vi "SemiProbe.vi"() -> ()   [LabVIEW 2019, in "SemiProbe.lvclass"]
uses:
  SemiProbe.lvclass
panel:
  in  "SemiProbe Probestation configuration":T1={"SP Local"=FALSE, "SP Min Usable Z"=0.0, "SP REMOTE Comm Parameters"={"SemiProbe VISA"="", "write delay(ms)"=500, "buffer is full loop multiplicity"=10, "read threshold check rate (ms)"=50}, "SP Comm Params"={"LF as Return EOL"=TRUE, "SP Error Debug"=FALSE}, "SP LOCAL Comm Parameters"={"address"="localhost", "port"=5050, "SP TCP Cnx ID"=refnum, "mode (standard)"=enum."Immediate", "bytes to read"=300, "timeout (ms)"=1000000}, "SP Operation Parameters"={"SP Load Less Than Thr?"=TRUE, "SP Load Threshold (um)"=4800.0, "SP Current Location"={"X (um)"=20.0, "Y (um)"=20.0, "Z (um)"=20.0, "T (degree)"=20.0}, "SP Chuck Speeds"={"XY Speed (10-100%)"=10.0, "Z Speed (10-100%)"=10.0, "T Speed (10-100%)"=10.0}, "Manual Step Parameters"={"Step in X"=FALSE, "X S-Speed [µm/step]"=5.0, "Step in Y"=FALSE, "Y S-Speed [µm/step]"=5.0, "Step in Z"=FALSE, "Z S-Speed [µm/step]"=5.0, "Step in T"=FALSE, "T S-Speed [mdegree/step]"=5.0, "X Increase"=TRUE, "Y Increase?"=TRUE, "Z Increase?"=TRUE, "T Increase?"=TRUE}, "Z Stepper"={"UP/DOWN"=FALSE, "UP/DOWN Speed [µm/step]"=20, "SP Z Step"=FALSE}, "Z Heights Set"=FALSE, "SP Contact Search"={"Contact Circuit"=enum."1", "Speed [1000-10000]"=1000.0, "Start Height [µm]"=0.0, "Search Band [µm]"=100.0, "Overdrive [µm]"=30.0}, "Separation Distance [µm]"=0, "Contact Height [µm]"=0, "Use Overdrive?"=FALSE, "Touchdown method"=enum."no feedback", "Arduino Edgesense params"={"touchdown height [µm]"=0, "search band [µm]"=100, "speed [µm/step]"=10, "overdrive [µm]"=30}}} {"SP Operation Parameters"."SP Contact Search"."Speed [1000-10000]" min=1000 max=10000; "SP Operation Parameters"."SP Load Threshold (um)" format="%#_6f"}
  # "Of value set in the SP Navigation panel."
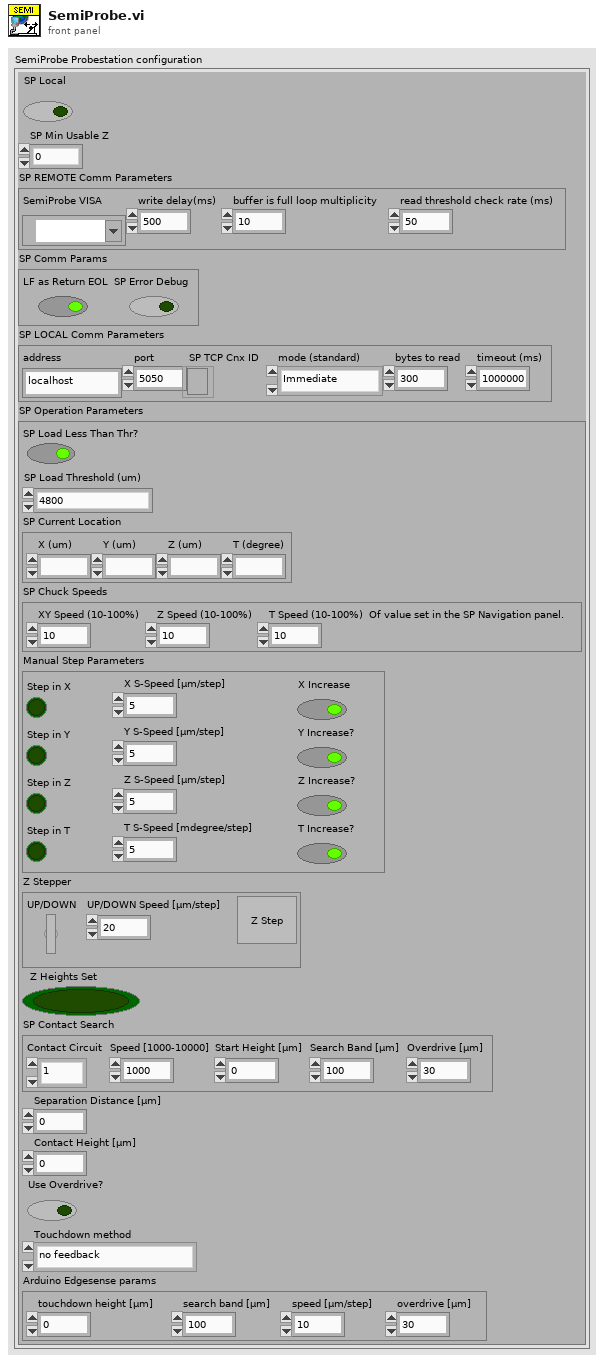
[diagram p1: front panel]
types:
  T1 = cluster{"SP Local":bool, "SP Min Usable Z":dbl, "SP REMOTE Comm Parameters":cluster{"SemiProbe VISA":refnum<visa-resource-name>, "write delay(ms)":i32, "buffer is full loop multiplicity":i32, "read threshold check rate (ms)":u32}, "SP Comm Params":cluster{"LF as Return EOL":bool, "SP Error Debug":bool}, "SP LOCAL Comm Parameters":cluster{"address":string, "port":i32, "SP TCP Cnx ID":refnum<k5>, "mode (standard)":enum16{"Standard", "Buffered", "CRLF", "Immediate"}, "bytes to read":i32, "timeout (ms)":i32}, "SP Operation Parameters":cluster{"SP Load Less Than Thr?":bool, "SP Load Threshold (um)":dbl, "SP Current Location":cluster{"X (um)":ext, "Y (um)":ext, "Z (um)":ext, "T (degree)":ext}, "SP Chuck Speeds":cluster{"XY Speed (10-100%)":dbl, "Z Speed (10-100%)":dbl, "T Speed (10-100%)":dbl}, "Manual Step Parameters":cluster{"Step in X":bool, "X S-Speed [µm/step]":sgl, "Step in Y":bool, "Y S-Speed [µm/step]":sgl, "Step in Z":bool, "Z S-Speed [µm/step]":sgl, "Step in T":bool, "T S-Speed [mdegree/step]":sgl, "X Increase":bool, "Y Increase?":bool, "Z Increase?":bool, "T Increase?":bool}, "Z Stepper":cluster{"UP/DOWN":bool, "UP/DOWN Speed [µm/step]":i32, "SP Z Step":bool}, "Z Heights Set":bool, "SP Contact Search":cluster{"Contact Circuit":enum16{"12", "1", "2"}, "Speed [1000-10000]":sgl, "Start Height [µm]":sgl, "Search Band [µm]":sgl, "Overdrive [µm]":sgl}, "Separation Distance [µm]":u32, "Contact Height [µm]":u32, "Use Overdrive?":bool, "Touchdown method":enum16{"no feedback", "Arduino edgesense", "SP contact circuit"}, "Arduino Edgesense params":cluster{"touchdown height [µm]":i32, "search band [µm]":u32, "speed [µm/step]":u32, "overdrive [µm]":u32}}}
diagram:
